vi "OneShot.vi"(11 "Input":bool) -> (3 "Pulse":bool)   [LabVIEW 2016]
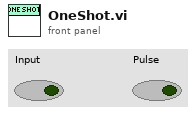
[diagram p1: front panel]
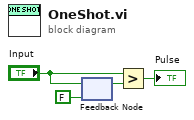
[diagram p0: block diagram]
diagram:
  n1 = feedback-in #1("Input") -> ()
  n2 = feedback #1(FALSE ("Input")) -> (w4:bool)
  n3 = Greater?(x="Input", y=w4) -> (0:→"Pulse":bool)
